vi "Keithley2400series_s2x2.vi"() -> ()   [LabVIEW 2014]
uses:
  <vilib>/Utility/file.llb/Write To Spreadsheet File (string).vi
panel:
  in  "Независимое упр.":bool
  in  "+ИП2":bool
  in  "VISA resource name2":refnum<visa-resource-name>
  out "SEEcount 2":dbl
  in  "SEE_th 2":dbl format="%.2f"
  out "Meas 2":dbl format="%#.6g"
  in  "Режим ИП 2  (0: Voltage)":u16(ring) items=["Voltage", "Current"]
  in  "Ограничение ИП2":dbl format="%.2f"
  in  "Выход ИП2":dbl
  out "SEEcount 1":dbl
  in  "SEE_th 1":dbl format="%.2f"
  out "Meas 1":dbl format="%#.6g"
  in  "stop":bool
  in  "Режим ИП1 (0: Voltage)":u16(ring) items=["Voltage", "Current"]
  in  "VISA resource name 1":refnum<visa-resource-name>
  in  "Serial Configuration":T1={"Baud Rate"=9600, "Parity"=0, "Data Bits"=8, "Stop Bits"=10, "Flow Control"=0} {"Flow Control" items=["None", "XON/XOFF", "RTS/CTS", "XON/XOFF & RTS/CTS", "DTR/DSR", "XON/XOFF & DTR/DSR"]; "Stop Bits" items=["1.0"=10, "1.5"=15, "2.0"=20]; "Data Bits" items=["7"=7, "8"=8]; "Parity" items=["None", "Odd", "Even", "Mark", "Space"]; "Baud Rate" items=["300"=300, "600"=600, "1200"=1200, "2400"=2400, "4800"=4800, "9600"=9600, "19200"=19200]}
  in  "Файл записи замеров":path
  in  "Ограничение ИП1":dbl format="%.2f"
  in  "Выход ИП1":dbl
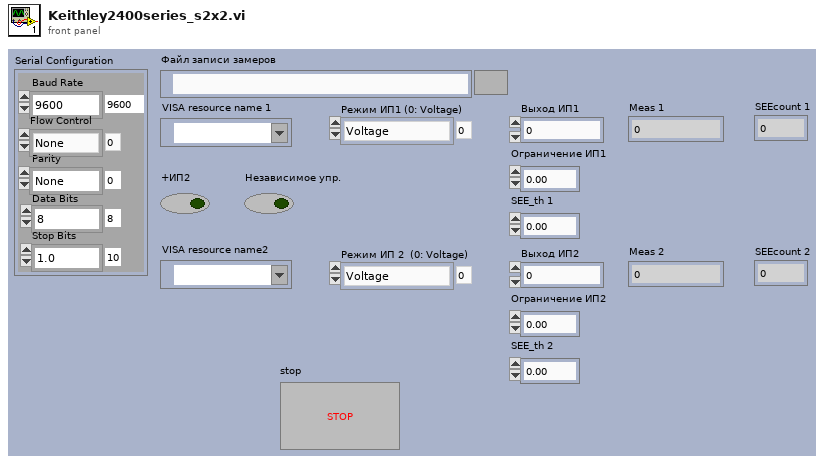
[diagram p1: front panel]
types:
  T1 = cluster{"Baud Rate":u32, "Parity":u16, "Data Bits":u16, "Stop Bits":u16, "Flow Control":u16}
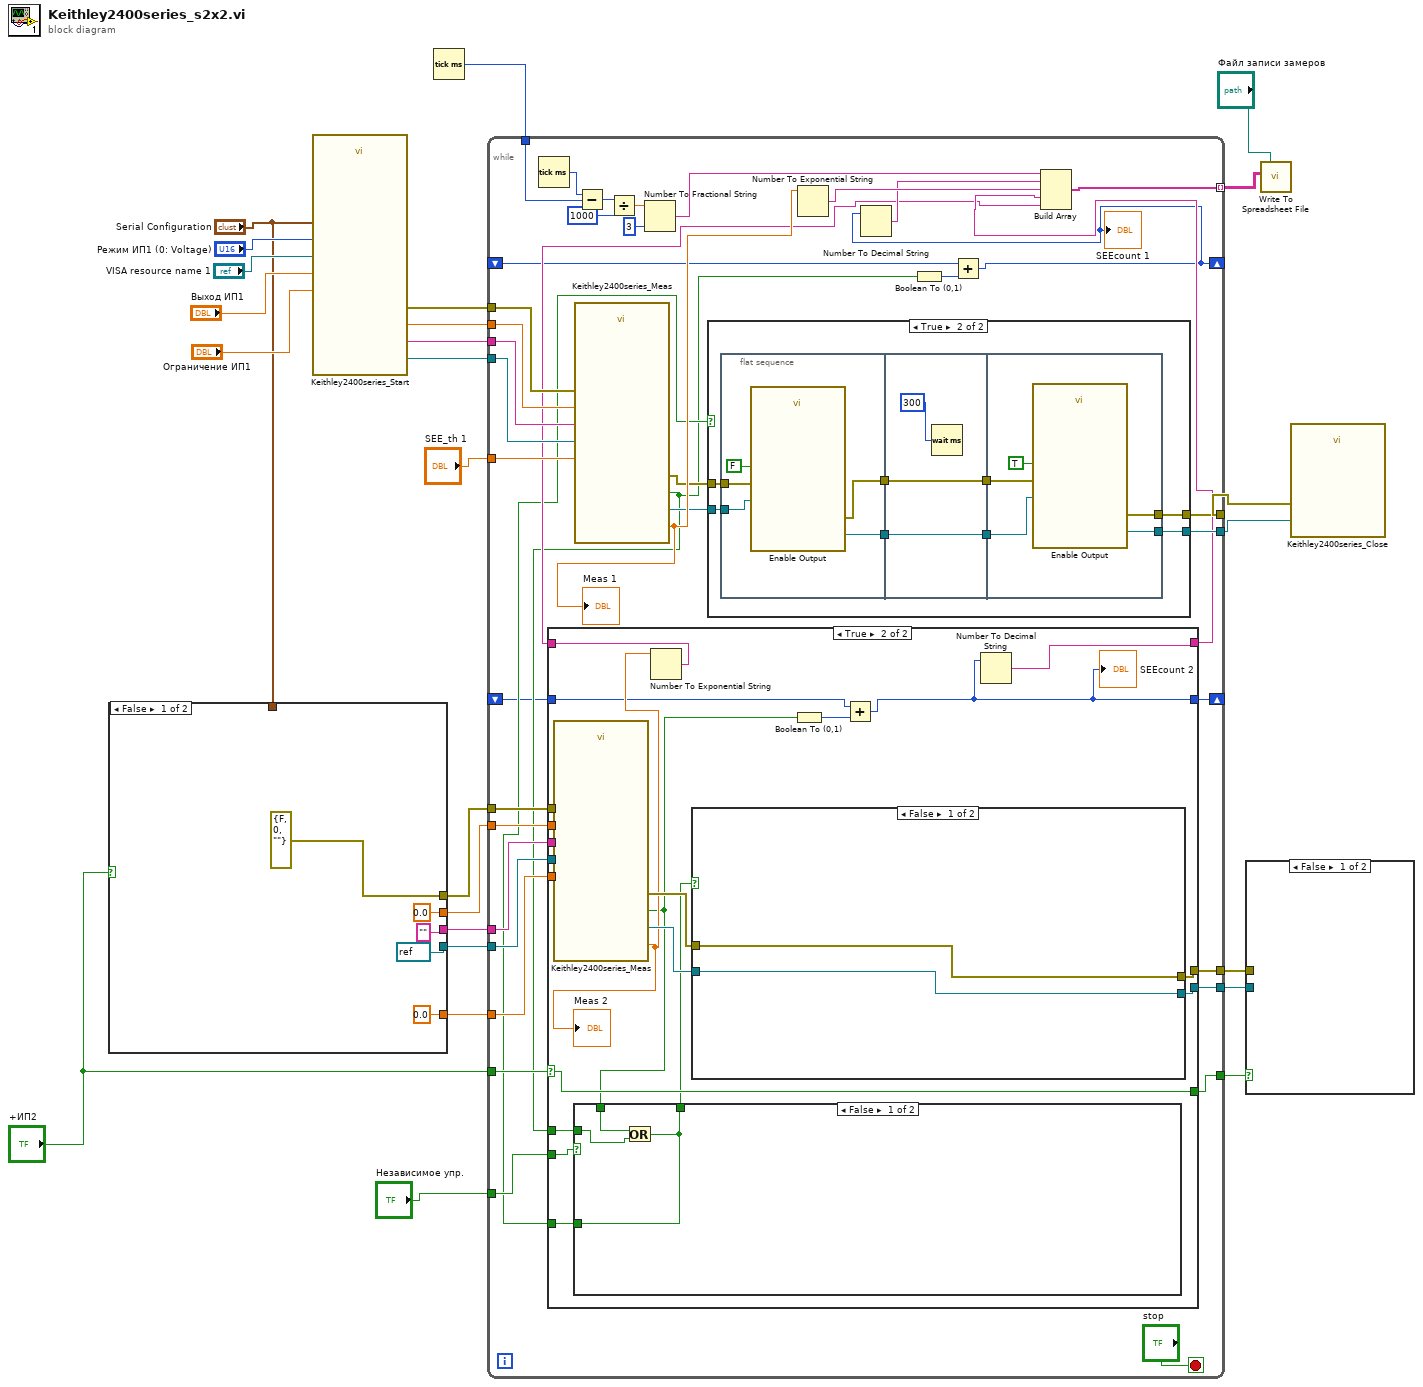
[diagram p0: block diagram]
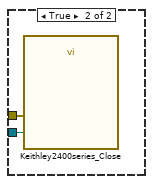
[diagram p2: hidden frame]
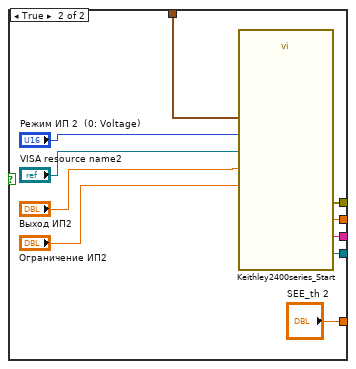
[diagram p3: hidden frame]
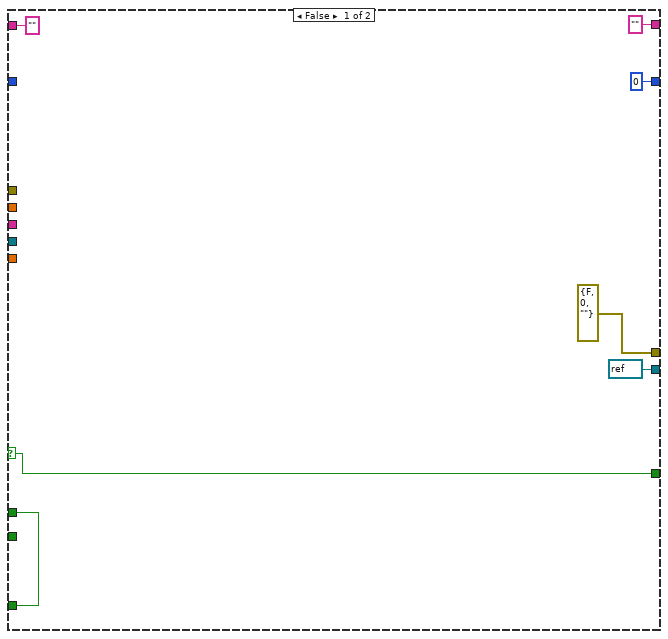
[diagram p4: hidden frame]
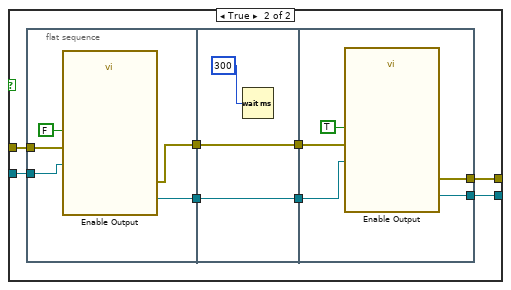
[diagram p6: hidden frame]
diagram:
  n1 = case shown="False" "+ИП2" {
    tunnel: "Serial Configuration" -> [_ w40]
    tunnel: [0.0 ("SEE_th 2") "SEE_th 2"] -> w10
    tunnel: [refnum<visa-resource-name> refnum ("VISA resource name out") w34] -> w9
    tunnel: ["" ("MEAS:Out") w33] -> w8
    tunnel: [0.0 ("MEAS mode 0,Volt") w32] -> w7
    tunnel: [errorcluster {"status"=FALSE, "code"=0, "source"=""} ("error out") w31] -> w6
    frame False {
    }
    frame True {
      n2 = call "Keithley2400series_Start.vi"("Serial Configuration"=w40, "Source Mode  (0: Voltage) 2"="Режим ИП 2  (0: Voltage)", "Ограничение"="Ограничение ИП2", "Выход"="Выход ИП2", "VISA resource name"="VISA resource name2") -> ("error out"=w31:errorcluster, "MEAS:Out"=w33:string, "MEAS mode 0,Volt"=w32:dbl, "VISA resource name out"=w34:refnum<visa-resource-name>)
    }
  }
  n3 = call "Keithley2400series_Start.vi"("Serial Configuration"="Serial Configuration", "Source Mode  (0: Voltage) 2"="Режим ИП1 (0: Voltage)", "Ограничение"="Ограничение ИП1", "Выход"="Выход ИП1", "VISA resource name"="VISA resource name 1") -> ("error out"=w20:errorcluster, "MEAS:Out"=w18:string, "MEAS mode 0,Volt"=w19:dbl, "VISA resource name out"=w17:refnum<visa-resource-name>)
  n4 = Tick Count (ms)() -> (millisecond timer value=w21:u32)
  n5 = while {
    tunnel: w21 -> [w76]
    tunnel: w20 -> [w64]
    tunnel: w19 -> [w65]
    tunnel: w18 -> [w66]
    tunnel: w17 -> [w67]
    tunnel: [w56] -> w16 mode=indexing
    tunnel: "SEE_th 1" -> [w72]
    tunnel: [w69] -> w14
    tunnel: [w68] -> w13
    shift-right: [w44] -> _
    shift-left: _ -> [w45]
    tunnel: w10 -> [w61]
    tunnel: w9 -> [w60]
    tunnel: w8 -> [w59]
    tunnel: w7 -> [w58]
    tunnel: w6 -> [w57]
    shift-right: [w43] -> _
    shift-left: _ -> [w42]
    tunnel: [w53] -> w5
    tunnel: [w52] -> w4
    tunnel: "+ИП2" -> [w51]
    tunnel: [w50] -> w2
    tunnel: "Независимое упр." -> [w49]
    stop <- "stop" stop-if-true
    n6 = Tick Count (ms)() -> (millisecond timer value=w80:u32)
    n7 = call "Keithley2400series_Meas.vi"("MEAS:<f>"=w66, "error in (no error)"=w64, "MEAS mode, 0 Volt"=w65, "ОРЭ_th"=w72, "VISA resource name in"=w67) -> ("error out"=w70:errorcluster, "SEE"=w46:bool, "Замер"=w73:dbl, "VISA out"=w71:refnum<visa-resource-name>)
    "Meas 1" <- w73
    n8 = case shown="True" w51 {
      selector: w51 -> [w83 w96]
      tunnel: w61 -> [_ w108]
      tunnel: w60 -> [_ w107]
      tunnel: w59 -> [_ w106]
      tunnel: w58 -> [_ w105]
      tunnel: w57 -> [_ w104]
      tunnel: ["" w97] -> w55
      tunnel: ["" w100] -> w54
      tunnel: [errorcluster {"status"=FALSE, "code"=0, "source"=""} ("error out") w99] -> w53
      tunnel: [refnum<visa-resource-name> refnum ("VISA resource name out") w98] -> w52
      tunnel: [w83 w96] -> w50
      tunnel: w49 -> [_ w95]
      tunnel: w46 -> [w82 w93]
      tunnel: [w82 w92] -> w48
      tunnel: [i16 0 w88] -> w43
      tunnel: w42 -> [_ w89]
      frame False {
      }
      frame True {
        n9 = call "Keithley2400series_Meas.vi"("MEAS:<f>"=w106, "error in (no error)"=w104, "MEAS mode, 0 Volt"=w105, "ОРЭ_th"=w108, "VISA resource name in"=w107) -> ("error out"=w103:errorcluster, "SEE"=w90:bool, "Замер"=w101:dbl, "VISA out"=w102:refnum<visa-resource-name>)
        "Meas 2" <- w101
        n10 = case shown="False" w95 {
          tunnel: [w109 w113] -> w94
          tunnel: w90 -> [w111 w113]
          tunnel: w93 -> [w110 w112]
          tunnel: [w109 w112] -> w92
          frame False {
            n11 = Or(x=w111, y=w110) -> (x .or. y?=w109:bool)
          }
          frame True {
          }
        }
        n12 = Number To Exponential String(number=w101) -> (E-format string=w100:string)  [unwired: 3 in]
        n13 = case shown="False" w94 {
          tunnel: w102 -> [w115 w123]
          tunnel: w103 -> [w114 w122]
          tunnel: [w114 w117] -> w99
          tunnel: [w115 w116] -> w98
          frame False {
          }
          frame True {
            n14 = flat-sequence {
              tunnel: w123 -> [w127]
              tunnel: w122 -> [w126]
              tunnel: [w125] -> w120
              tunnel: [w124] -> w118
              tunnel: [w130] -> w121
              tunnel: w120 -> [w130]
              tunnel: [w129] -> w119
              tunnel: w118 -> [w129]
              tunnel: w121 -> [w135]
              tunnel: w119 -> [w134]
              tunnel: [w133] -> w117
              tunnel: [w132] -> w116
              frame #0 {
                n15 = call "Enable Output.vi"("error in (no error)"=w126, "Enable Output (T: Enable)"=FALSE, "VISA resource name"=w127) -> ("error out"=w125:errorcluster, "VISA resource name out"=w124:refnum<visa-resource-name>)  [unwired: 7 in]
              }
              frame #1 {
                n16 = Wait (ms)(milliseconds to wait=u32 300) -> ()  [unwired: 1 out]
              }
              frame #2 {
                n17 = call "Enable Output.vi"("error in (no error)"=w135, "Enable Output (T: Enable)"=TRUE, "VISA resource name"=w134) -> ("error out"=w133:errorcluster, "VISA resource name out"=w132:refnum<visa-resource-name>)  [unwired: 7 in]
              }
            }
          }
        }
        n18 = Boolean To (0,1)(Boolean=w90) -> (0, 1=w91:i16)
        n19 = Add(x=w89, y=w91) -> (x+y=w88:i16)
        "SEEcount 2" <- w88
        n20 = Number To Decimal String(number=w88) -> (decimal integer string=w97:string)  [unwired: 1 in]
      }
    }
    n21 = Subtract(x=w80, y=w76) -> (x-y=w79:u32)
    n22 = Divide(x=w79, y=u32 1000) -> (x/y=w77:dbl)
    n23 = Number To Fractional String(number=w77, precision (6)=i16 3) -> (F-format string=w75:string)  [unwired: 2 in]
    n24 = case shown="True" w48 {
      tunnel: w71 -> [w138 w146]
      tunnel: w70 -> [w137 w145]
      tunnel: [w137 w140] -> w69
      tunnel: [w138 w139] -> w68
      frame False {
      }
      frame True {
        n25 = flat-sequence {
          tunnel: w146 -> [w150]
          tunnel: w145 -> [w149]
          tunnel: [w148] -> w143
          tunnel: [w147] -> w141
          tunnel: [w153] -> w144
          tunnel: w143 -> [w153]
          tunnel: [w152] -> w142
          tunnel: w141 -> [w152]
          tunnel: w144 -> [w158]
          tunnel: w142 -> [w157]
          tunnel: [w156] -> w140
          tunnel: [w155] -> w139
          frame #0 {
            n26 = call "Enable Output.vi"("error in (no error)"=w149, "Enable Output (T: Enable)"=FALSE, "VISA resource name"=w150) -> ("error out"=w148:errorcluster, "VISA resource name out"=w147:refnum<visa-resource-name>)  [unwired: 7 in]
          }
          frame #1 {
            n27 = Wait (ms)(milliseconds to wait=u32 300) -> ()  [unwired: 1 out]
          }
          frame #2 {
            n28 = call "Enable Output.vi"("error in (no error)"=w158, "Enable Output (T: Enable)"=TRUE, "VISA resource name"=w157) -> ("error out"=w156:errorcluster, "VISA resource name out"=w155:refnum<visa-resource-name>)  [unwired: 7 in]
          }
        }
      }
    }
    n29 = Number To Exponential String(number=w73) -> (E-format string=w63:string)  [unwired: 3 in]
    n30 = Boolean To (0,1)(Boolean=w46) -> (0, 1=w47:i16)
    n31 = Add(x=w45, y=w47) -> (x+y=w44:i16)
    "SEEcount 1" <- w44
    n32 = Number To Decimal String(number=w44) -> (decimal integer string=w62:string)  [unwired: 1 in]
    n33 = Build Array(w75, w62, w63, w55, w54) -> (w56:string[])
  }
  n34 = case shown="False" w2 {
    tunnel: w5 -> [_ w161]
    tunnel: w4 -> [_ w160]
    frame False {
    }
    frame True {
      n35 = call "Keithley2400series_Close.vi"("error in (no error)"=w161, "VISA resource name"=w160) -> ()
    }
  }
  n36 = call-poly <vilib>:"Write To Spreadsheet File.vi"("2D data"=w16, "file path (dialog if empty)"="Файл записи замеров") -> ()  [unwired: 6 in, 1 out]
  n37 = call "Keithley2400series_Close.vi"("error in (no error)"=w14, "VISA resource name"=w13) -> ()
